vi "TC560-Resistance Range.vi"(8 "error in":errorcluster, 10 "Range":enum16{"30mOHM", "300mIHM", "3OHM", "AUTO"}(ring), 11 "VISA Resource Name In":refnum<visa-resource-name>) -> (0 "error out":errorcluster, 3 "VISA Resource Name Out":refnum<visa-resource-name>)   [LabVIEW 2018]
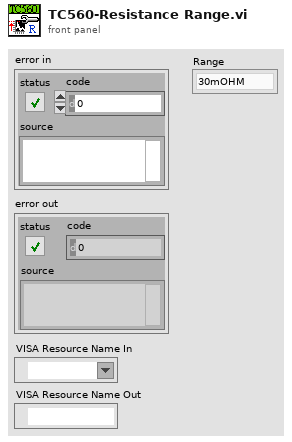
[diagram p1: front panel]
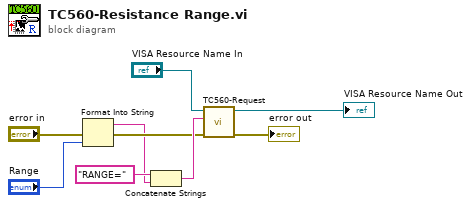
[diagram p0: block diagram]
diagram:
  n1 = Format Into String(error in="error in", "Range") -> (resulting string=w2:string, error out=w4:errorcluster)  [unwired: 2 in]
  n2 = Concatenate Strings("RANGE=" ("write buffer"), w2) -> (w7:string)
  n3 = call "TC560-Request.vi"("error in"=w4, "Command"=w7, "VISA Resource Name In"="VISA Resource Name In") -> ("error out"=→"error out":errorcluster, "VISA Resource Name Out"=→"VISA Resource Name Out":refnum<visa-resource-name>)  [unwired: 6 in, 1 out]
